vi "Teleop.vi"(10 "Match Info":T1={"Autonomous Elapsed Seconds"=0.0, "TeleOp Elapsed Seconds"=0.0, "Disabled Elapsed Seconds"=0.0, "Visited Autonomous"=FALSE, "Visited TeleOp"=FALSE, "Visited Disabled"=FALSE, "Autonomous Settings"={"Autonomous Style"=enum."Independent", "VI Refnum"=refnum}}, 11 "Call Context":T2) -> ()   [LabVIEW 2016]
doc: "This VI is called for each TeleOp packet received from the DS where the robot is not disabled. It is often used to read from the joysticks and update I/O or to update setpoints for timed control loops. It should complete and return within 20 milliseconds or it may miss DS packets."
uses:
  <vilib>/Rock Robotics/WPI/DriverStation/WPI_DriverStationDerivedRobotMode.ctl
  <vilib>/Rock Robotics/WPI/DriverStation/WPI_DriverStationMatch Info.ctl
  <vilib>/Rock Robotics/WPI/Solenoid/WPI_SolenoidValue.ctl
  <vilib>/Rock Robotics/WPI/Utilities/WPI_GetSetVariantRefNum.vi
  <vilib>/Rock Robotics/WPI/Solenoid/WPI_SolenoidSetEnum.vi
panel:
  in  "reset gyro":bool
  out "Angle":dbl
  in  "Range":dbl=25.0 format="%#_13g"
  out "Encoder Position R":dbl
  out "Encoder Position L":dbl
  out "Gyro Angle":dbl format="%#_13g"
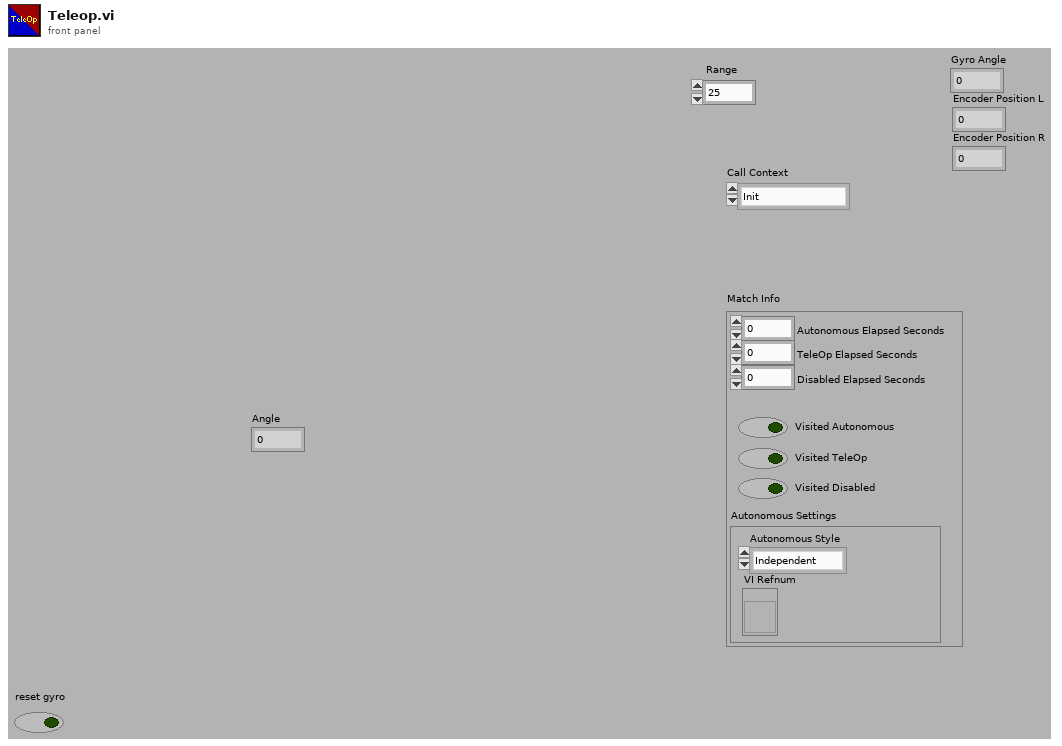
[diagram p1: front panel]
types:
  T1 = typedef "WPI_DriverStationMatch Info.ctl" = cluster{"Autonomous Elapsed Seconds":dbl, "TeleOp Elapsed Seconds":dbl, "Disabled Elapsed Seconds":dbl, "Visited Autonomous":bool, "Visited TeleOp":bool, "Visited Disabled":bool, "Autonomous Settings":cluster{"Autonomous Style":enum16{"Iterative", "Independent"}, "VI Refnum":refnum<vi>}}
  T2 = typedef "WPI_DriverStationDerivedRobotMode.ctl" = enum16{"Init", "Execute", "Stop"}
  T3 = typedef "WPI_SolenoidValue.ctl" = enum16{"Off", "On", "Forward", "Reverse"}
  T4 = typedef "WPI_GyroDevRef.ctl" = cluster{"DevStatus":errorcluster, "Analog Channel":T5, "Offset":dbl, "Gain (VoltsPerDegree/Second)":dbl, "Gyro Type":enum16{"Analog", "XRS450"}, "Handle":i32, "SPI Bus":T6, "Device Found":bool, "Sample Rate":dbl, "Calibrate On Open":bool}
  T5 = typedef "FPGA_AIChannel.ctl" = enum8{"AI 0", "AI 1", "AI 2", "AI 3", "AI MXP 0", "AI MXP 1", "AI MXP 2", "AI MXP 3", "Invalid"}
  T6 = typedef "spi_bus.ctl" = enum16{"SPI On-Board, CS0", "SPI On-Board, CS1", "SPI On-Board, CS2", "SPI On-Board, CS3", "SPI MXP", "Invalid"}
  T7 = typedef "WPI_JoystickDevRef.ctl" = cluster{"Device":T8}
  T8 = typedef "WPI_JoystickDeviceEnum.ctl" = enum16{"USB 0", "USB 1", "USB 2", "USB 3", "USB 4", "USB 5"}
  T9 = typedef "WPI_MotorControlDeviceRef.ctl" = cluster{"DeviceStatus":errorcluster, "Type":T10, "PWM":cluster{"PWM Channel":T11, "DeadBand":T12}, "CAN":cluster{"Device Number":u8, "SetOutput VI Ref":variant, "GetOutput VI Ref":variant, "Enable VI Ref":variant, "Disable VI Ref":variant, "Data":variant}, "Invert":bool}
  T10 = typedef "WPI_MotorControlType.ctl" = enum16{"PWM", "CAN"}
  T11 = typedef "FPGA_DIOPWMChannel.ctl" = enum8{"PWM 0", "PWM 1", "PWM 2", "PWM 3", "PWM 4", "PWM 5", "PWM 6", "PWM 7", "PWM 8", "PWM 9", "PWM MXP 0", "PWM MXP 1", "PWM MXP 2", "PWM MXP 3", "PWM MXP 4", "PWM MXP 5", "PWM MXP 6", "PWM MXP 7", "PWM MXP 8", "PWM MXP 9", "Invalid"}
  T12 = typedef "WPI_PWMDeadband.ctl" = cluster{"Name":string, "maxPositivePwm":i32, "minPositivePwm":i32, "centerPwm":i32, "maxNegativePwm":i32, "minNegativePwm":i32, "angularRange":u16}
  T13 = typedef "WPI_CANTalonSRX_GlobalStatus.ctl" = cluster{"Applied Throttle":dbl, "Module Enabled":bool, "CAN Error":errorcluster, "Closed Loop Error":dbl, "Forward Limit Switch Closed":bool, "Reverse Limit Switch Closed":bool, "Sensor Position":dbl, "Sensor Velocity":dbl, "Current":dbl, "Sticky Fault - Over Temp":bool, "Sticky Fault - Under Voltage":bool, "Sticky Fault - Forward Limit":bool, "Sticky Fault - Reverse Limit":bool, "Sticky Fault - Forward Soft Limit":bool, "Sticky Fault - Reverse Soft Limit":bool, "Brake is Enabled":bool, "Encoder Position":dbl, "Encoder Velocity":dbl, "Encoder Index Count":dbl, "Encoder A Pin State":bool, "Encoder B Pin State":bool, "Encoder Index Pin State":bool, "Analog In":dbl, "Analog In Velocity":dbl, "Temperature (C)":dbl, "Battery Voltage":dbl, "Control 5 Is Supported":bool, "Current Profile Slot Select":dbl, "Pos Div 8":bool, "Vel Div 4":bool, "Pulse Width Position":i32, "Pulse Width Velocity":i32, "Pulse Width Rise To Rise (us)":i32, "Pulse Width Rise To Fall (us)":i32, "Mot Prof Active Is Under Run":bool, "Mot Prof Active Has Under Run":bool, "Mot Prof Active Is Last":bool, "Mot Prof Active Velocity Only":bool, "Mot Prof Active Is Valid":bool, "Mot Prof Buffer Is Full":bool, "Mot Prof Active Profile Slot Select":i32, "Mot Prof NextID":i32, "Mot Prof Count":i32, "Mot Prof Active Velocity":dbl, "Mot Prof Active Position":dbl, "Mot Prof Output Enable":i32}
  T14 = typedef "WPI_SolenoidDevRef.ctl" = cluster{"DevStatus":errorcluster, "Pneumatics Control Module":u8, "Forward Solenoid Channel":T15, "Reverse Solenoid Channel":T15}
  T15 = typedef "WPI_SolenoidChannel.ctl" = enum8{"Solenoid 0", "Solenoid 1", "Solenoid 2", "Solenoid 3", "Solenoid 4", "Solenoid 5", "Solenoid 6", "Solenoid 7", "Invalid"}
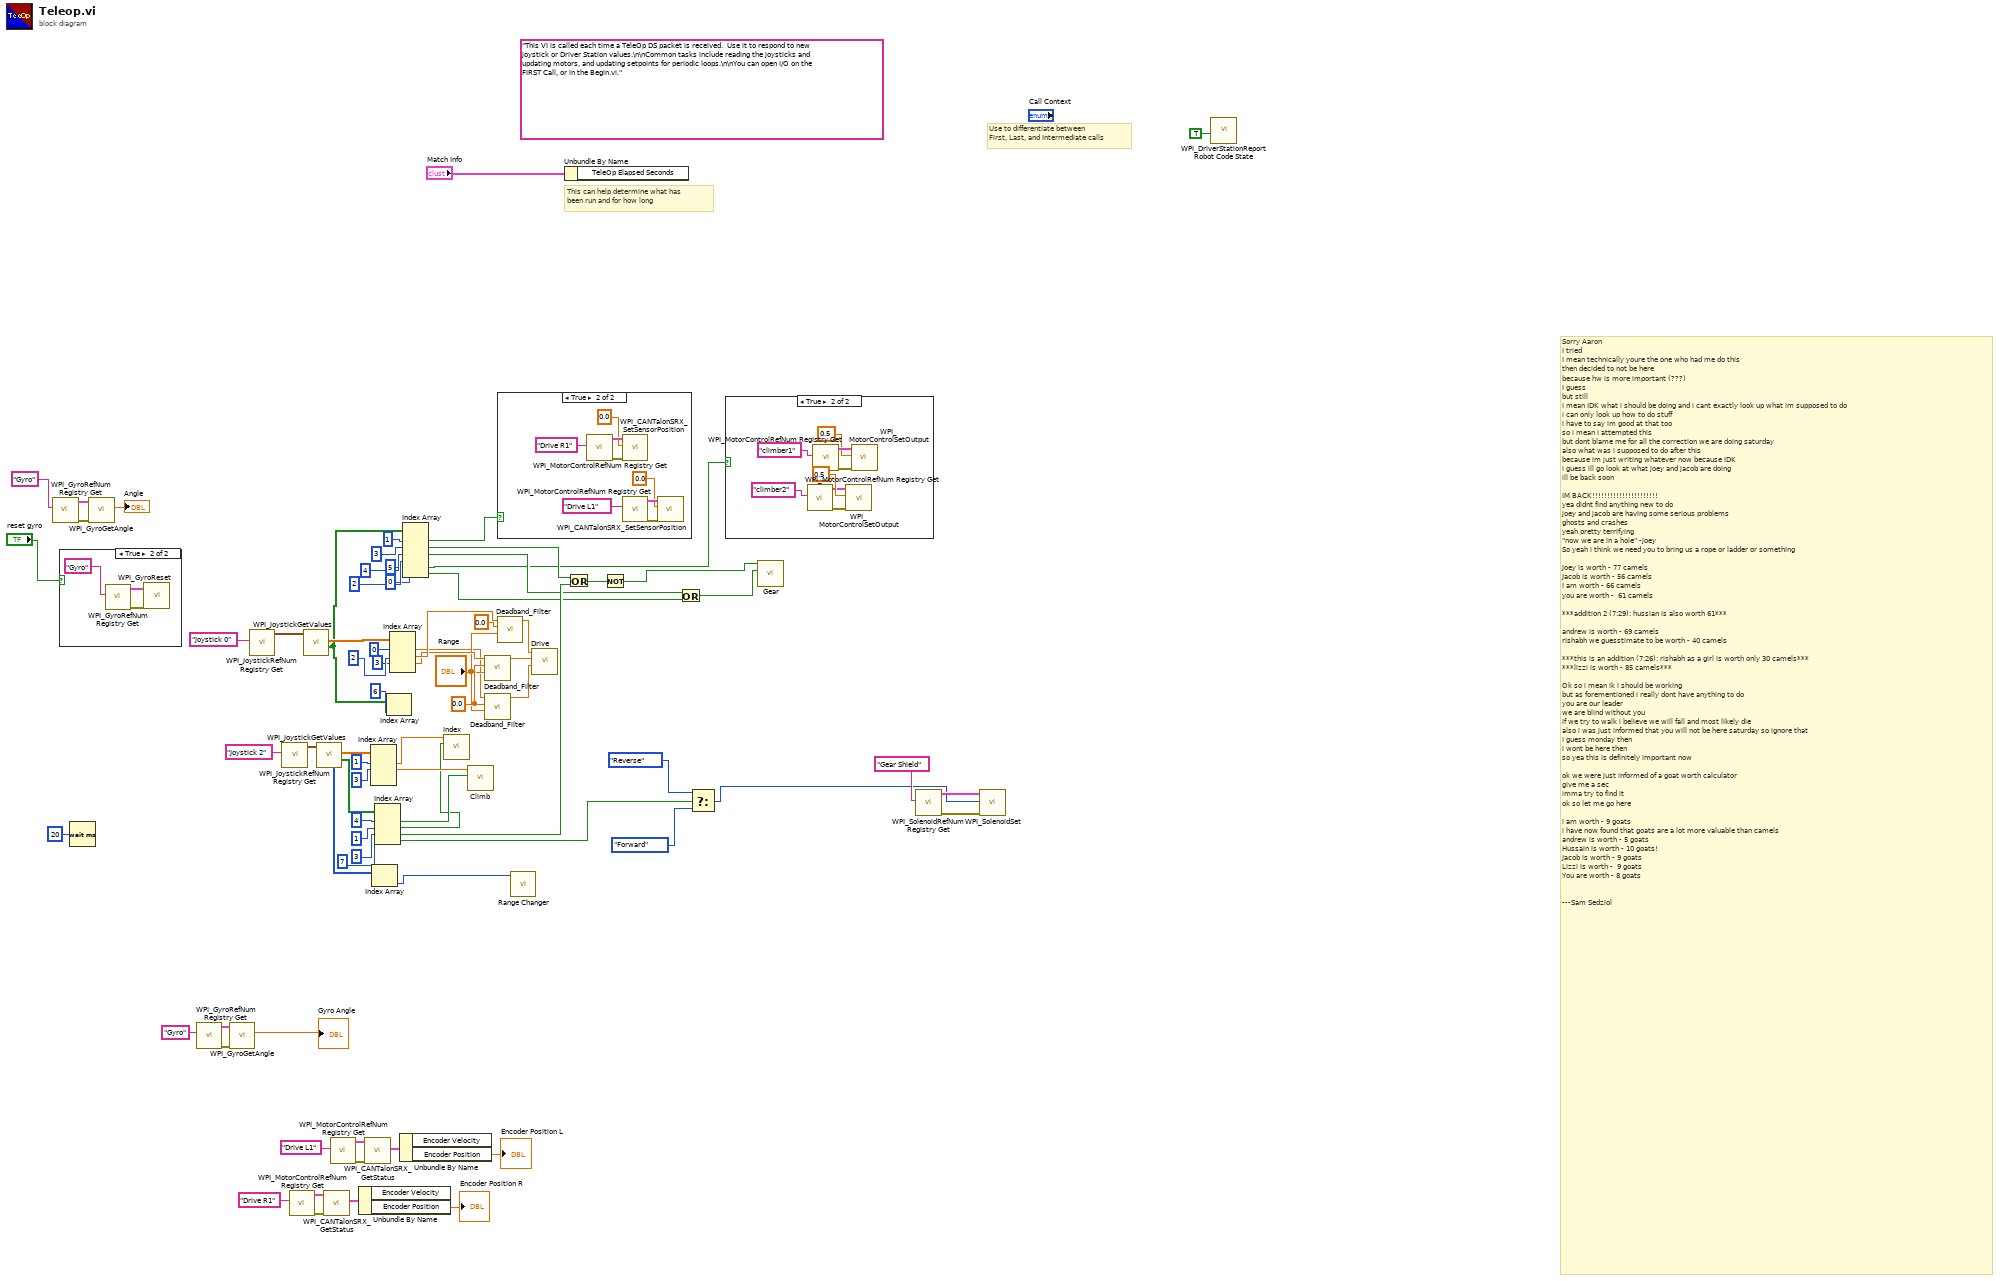
[diagram p0: block diagram]
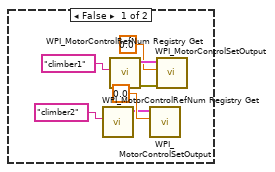
[diagram p3: hidden frame]
diagram:
  w12 = 0.0 ("Target")
  (unwired) "This VI is called each time a TeleOp DS packet is received.  Use it to respond to new joystick or Driver Station values.\n\nCommon tasks include reading the joysticks and updating motors, and updating setpoints for periodic loops.\n\nYou can open I/O on the FIRST Call, or in the Begin.vi."
  # "Sorry Aaron\nI tried\nI mean technically youre the one who had me do this\nthen decided to not be here\nbecause hw is more important (???)\nI guess\nbut still\nI mean IDK what i should be doing and i cant exactly look up what im supposed to do\ni can only look up how to do stuff\ni have to say im good at that too\nso i mean i attempted this\nbut dont blame me for all the correction we are doing saturday\nalso what was i supposed to do after this\nbecause im just writing whatever now because IDK\ni guess ill go look at what joey and jacob are doing\nill be back soon\n\nIM BACK!!!!!!!!!!!!!!!!!!!!!!\nyea didnt find anything new to do\njoey and jacob are having some serious problems\nghosts and crashes\nyeah pretty terrifying\n\"now we are in a hole\" -joey\nSo yeah i think we need you to bring us a rope or ladder or something\n\nJoey is worth - 77 camels\nJacob is worth - 56 camels\nI am worth - 66 camels\nyou are worth -  61 camels \n\n***addition 2 (7:29): hussian is also worth 61***\n\nandrew is worth - 69 camels\nrishabh we guesstimate to be worth - 40 camels\n\n***this is an addition (7:26): rishabh as a girl is worth only 30 camels***\n***lizzi is worth - 85 camels***\n\nOk so i mean ik i should be working\nbut as forementioned i really dont have anything to do\nyou are our leader\nwe are blind without you\nif we try to walk i believe we will fall and most likely die\nalso i was just informed that you will not be here saturday so ignore that\ni guess monday then\ni wont be here then\nso yea this is definitely important now\n\nok we were just informed of a goat worth calculator\ngive me a sec \nimma try to find it\nok so let me go here\n\ni am worth - 9 goats\ni have now found that goats are a lot more valuable than camels\nandrew is worth - 5 goats\nHussain is worth - 10 goats! \nJacob is worth - 9 goats\nLizzi is worth -  9 goats\nYou are worth - 8 goats\n\n\n---Sam Sedziol"
  # "Use to differentiate between\nFirst, Last, and Intermediate calls"
  # "This can help determine what has\nbeen run and for how long"
  n1 = call <vilib>:"WPI_GyroRefNum Registry Get.vi"("refnum name"="Gyro") -> ("error out"=w5:errorcluster, "GyroDevRef"=w4:T4)  [unwired: 9 in]
  n2 = case shown="True" "reset gyro" {
    frame False {
    }
    frame True {
      n3 = call <vilib>:"WPI_GyroRefNum Registry Get.vi"("refnum name"="Gyro") -> ("error out"=w79:errorcluster, "GyroDevRef"=w78:T4)  [unwired: 9 in]
      n4 = call <vilib>:"WPI_GyroReset.vi"("error in"=w79, "GyroDevRef"=w78) -> ()  [unwired: 8 in, 2 out]
    }
  }
  n5 = Wait (ms)(milliseconds to wait=u32 20) -> ()  [unwired: 1 out]
  n6 = call <vilib>:"WPI_GyroGetAngle.vi"("error in"=w5, "GyroDevRef"=w4) -> ("Angle"=→"Angle":dbl)  [unwired: 5 in, 4 out]
  n7 = call <vilib>:"WPI_GyroRefNum Registry Get.vi"("refnum name"="Gyro") -> ("error out"=w59:errorcluster, "GyroDevRef"=w58:T4)  [unwired: 9 in]
  n8 = call <vilib>:"WPI_GyroGetAngle.vi"("error in"=w59, "GyroDevRef"=w58) -> ("Angle"=→"Gyro Angle":dbl)  [unwired: 5 in, 4 out]
  n9 = call <vilib>:"WPI_JoystickRefNum Registry Get.vi"("refnum name"="Joystick 0") -> ("JoystickDevRef"=w65:T7)  [unwired: 1 in, 9 out]
  n10 = call <vilib>:"WPI_JoystickRefNum Registry Get.vi"("refnum name"="Joystick 2") -> ("JoystickDevRef"=w72:T7)  [unwired: 1 in, 9 out]
  n11 = call <vilib>:"WPI_MotorControlRefNum Registry Get.vi"("refnum name"="Drive R1") -> ("error out"=w53:errorcluster, "MotorControlDevRef"=w54:T9)  [unwired: 9 in]
  n12 = call <vilib>:"WPI_JoystickGetValues.vi"("JoystickDevRef"=w65) -> ("Buttons"=w19:bool[], "Axes"=w74:dbl[])  [unwired: 6 in, 3 out]
  n13 = call <vilib>:"WPI_JoystickGetValues.vi"("JoystickDevRef"=w72) -> ("Buttons"=w70:bool[], "Axes"=w71:dbl[], "POVs"=w32:i16[])  [unwired: 6 in, 2 out]
  n14 = call <vilib>:"WPI_CANTalonSRX_GetStatus.vi"("error in (no error)"=w53, "CAN Talon SRX Ref"=w54) -> ("Talon SRX Status"=w51:T13)  [unwired: 7 in, 2 out]
  n15 = call <vilib>:"WPI_MotorControlRefNum Registry Get.vi"("refnum name"="Drive L1") -> ("error out"=w50:errorcluster, "MotorControlDevRef"=w55:T9)  [unwired: 9 in]
  n16 = Unbundle By Name(w51) -> ("Encoder Position"=→"Encoder Position R":dbl)  [unwired: 1 out]
  n17 = call <vilib>:"WPI_CANTalonSRX_GetStatus.vi"("error in (no error)"=w50, "CAN Talon SRX Ref"=w55) -> ("Talon SRX Status"=w52:T13)  [unwired: 7 in, 2 out]
  n18 = Index Array(array=w71, index #1=1 ("index"), index #2=3 ("index")) -> (element #1=w45:dbl, element #2=w66:dbl)  [unwired: 2 in, 2 out]
  n19 = Index Array(array=w32) -> (element=w31:i16)  [unwired: 1 in]
  n20 = Index Array(array=w70, index #1=4 ("index"), index #2=1 ("index"), index #3=3 ("index"), index #4=7) -> (element #1=w41:bool, element #2=w22:bool, element #3=w42:bool, element #4=w25:bool)
  n21 = Index Array(array=w19, index=6) -> ()  [unwired: 1 out]
  n22 = Index Array(array=w74, index #1=0 ("index"), index #2=2 ("index"), index #3=3 ("index")) -> (element #1=w8:dbl, element #2=w18:dbl, element #3=w11:dbl)  [unwired: 1 in, 1 out]
  n23 = Unbundle By Name(w52) -> ("Encoder Position"=→"Encoder Position L":dbl)  [unwired: 1 out]
  n24 = Index Array(array=w19, index #1=1 ("index"), index #2=3 ("index"), index #3=4 ("index"), index #4=2 ("index"), index #5=5 ("index"), index #6=0 ("index")) -> (element #1=w68:bool, element #2=w37:bool, element #3=w36:bool, element #5=w20:bool, element #6=w6:bool)  [unwired: 1 out]
  n25 = call "Index.vi"("Shoot"=w22, "Output"=w45) -> ()  [unwired: 10 in]
  n26 = call "Climb.vi"("Backwards?"=w41, "Effort"=w66) -> ()  [unwired: 10 in]
  n27 = call "Deadband_Filter.vi"("Range"="Range", "Target"=w12, "Joystick Input"=w11) -> ("Output"=w9:dbl)  [unwired: 8 in]
  n28 = call "Deadband_Filter.vi"("Range"="Range", "Target"=w12, "Joystick Input"=w8) -> ("Output"=w14:dbl)  [unwired: 8 in]
  n29 = case shown="True" w68 {
    frame False {
    }
    frame True {
      n30 = call <vilib>:"WPI_MotorControlRefNum Registry Get.vi"("refnum name"="Drive R1") -> ("error out"=w83:errorcluster, "MotorControlDevRef"=w82:T9)  [unwired: 9 in]
      n31 = call <vilib>:"WPI_CANTalonSRX_SetSensorPosition.vi"("error in (no error)"=w83, "New Sensor Position"=0.0, "CAN Talon SRX Ref"=w82) -> ()  [unwired: 7 in, 2 out]
      n32 = call <vilib>:"WPI_MotorControlRefNum Registry Get.vi"("refnum name"="Drive L1") -> ("error out"=w85:errorcluster, "MotorControlDevRef"=w86:T9)  [unwired: 9 in]
      n33 = call <vilib>:"WPI_CANTalonSRX_SetSensorPosition.vi"("error in (no error)"=w85, "New Sensor Position"=0.0, "CAN Talon SRX Ref"=w86) -> ()  [unwired: 7 in, 2 out]
    }
  }
  n34 = call "Deadband_Filter.vi"("Range"="Range", "Target"=0.0, "Joystick Input"=w18) -> ("Output"=w13:dbl)  [unwired: 8 in]
  n35 = call "Range Changer.vi"("POV"=w31) -> ()  [unwired: 10 in, 1 out]
  n36 = call "Drive.vi"("Joystick 1"=w14, "RT"=w9, "LT"=w13) -> ()  [unwired: 9 in]
  n37 = Unbundle By Name("Match Info") -> ()  [unwired: 1 out]
  n38 = Or(x=w37, y=w42) -> (x .or. y?=w60:bool)
  n39 = Not(x=w60) -> (.not. x?=w35:bool)
  n40 = Or(x=w36, y=w6) -> (x .or. y?=w34:bool)
  n41 = Select(t=WPI_SolenoidValue."Reverse" ("Value"), s=w25, f=WPI_SolenoidValue."Forward" ("Value")) -> (s? t:f=w23:T3)
  n42 = case shown="True" w20 {
    frame False {
      n43 = call <vilib>:"WPI_MotorControlRefNum Registry Get.vi"("refnum name"="climber2") -> ("MotorControlDevRef"=w90:T9)  [unwired: 9 in, 1 out]
      n44 = call <vilib>:"WPI_MotorControlRefNum Registry Get.vi"("refnum name"="climber1") -> ("error out"=w94:errorcluster, "MotorControlDevRef"=w93:T9)  [unwired: 9 in]
      n45 = call <vilib>:"WPI_MotorControlSetOutput.vi"("Output"=0.0, "MotorControlDevRef"=w90) -> ()  [unwired: 7 in, 3 out]
      n46 = call <vilib>:"WPI_MotorControlSetOutput.vi"("error in (no error)"=w94, "Output"=0.0, "MotorControlDevRef"=w93) -> ()  [unwired: 6 in, 3 out]
    }
    frame True {
      n47 = call <vilib>:"WPI_MotorControlRefNum Registry Get.vi"("refnum name"="climber2") -> ("error out"=w97:errorcluster, "MotorControlDevRef"=w98:T9)  [unwired: 9 in]
      n48 = call <vilib>:"WPI_MotorControlRefNum Registry Get.vi"("refnum name"="climber1") -> ("error out"=w102:errorcluster, "MotorControlDevRef"=w101:T9)  [unwired: 9 in]
      n49 = call <vilib>:"WPI_MotorControlSetOutput.vi"("error in (no error)"=w97, "Output"=0.5, "MotorControlDevRef"=w98) -> ()  [unwired: 6 in, 3 out]
      n50 = call <vilib>:"WPI_MotorControlSetOutput.vi"("error in (no error)"=w102, "Output"=0.5, "MotorControlDevRef"=w101) -> ()  [unwired: 6 in, 3 out]
    }
  }
  n51 = call "Gear.vi"("Gear0?"=w34, "Gear1?"=w35) -> ()  [unwired: 10 in]
  n52 = call <vilib>:"WPI_SolenoidRefNum Registry Get.vi"("refnum name"="Gear Shield") -> ("error out"=w28:errorcluster, "SolenoidDevRef"=w27:T14)  [unwired: 9 in]
  n53 = call-poly <vilib>:"WPI_SolenoidSet.vi"("error in (no error)"=w28, "Value"=w23, "SolenoidDevRef"=w27) -> ()  [unwired: 7 in, 2 out]
  n54 = call <vilib>:"WPI_DriverStationReport Robot Code State.vi"("TeleOp"=TRUE ("Autonomous")) -> ()  [unwired: 10 in, 1 out]
